vi "TDC_getSyncDivider.vi"(11 "Error In":errorcluster) -> (4 "Divider":i32, 6 "Reconstruct":bool, 15 "Error Out":errorcluster)   [LabVIEW 2011]
uses:
  tdcbase.dll
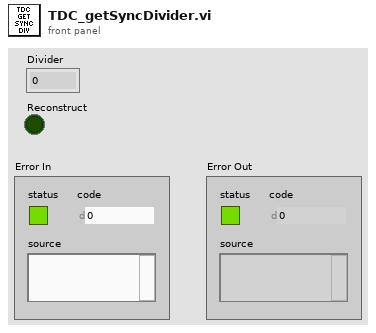
[diagram p1: front panel]
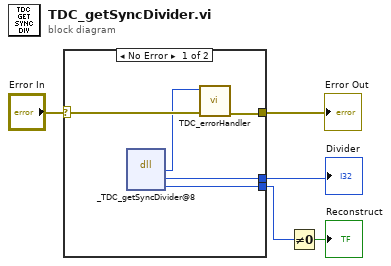
[diagram p0: block diagram]
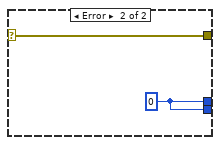
[diagram p2: hidden frame]
diagram:
  n1 = case shown="No Error" "Error In" {
    selector: "Error In" -> [w10 w12]
    tunnel: [w9 w12] -> w4
    tunnel: [w7 w11] -> w1
    tunnel: [w6 w11] -> w3
    frame No Error {
      n2 = dll-call lib="X:/tdcbase.dll" fn="_TDC_getSyncDivider@8"() -> ("return type"=w8:i32, "divider"=w6:i32, "Reconstruct"=w7:i32)  [unwired: 5 in, 2 out]
      n3 = call "TDC_errorHandler.vi"("Error In"=w10, "TDC Return Code"=w8) -> ("Error Out"=w9:errorcluster)  [unwired: 9 in]
    }
    frame Error {
      w11 = 0
    }
  }
  "Error Out" <- w4
  "Divider" <- w3
  n4 = Not Equal To 0?(x=w1) -> (x != 0?=→"Reconstruct":bool)
